vi "pop.vi"(0 "Buffer":string) -> (1 "New Buffer":string, 2 "Value":u8)   [LabVIEW 2022 SP3]
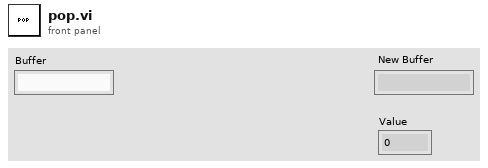
[diagram p1: front panel]
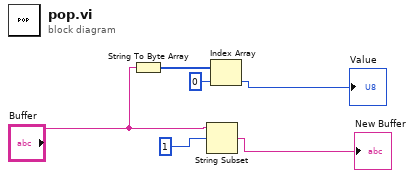
[diagram p0: block diagram]
diagram:
  n1 = String To Byte Array(string="Buffer") -> (unsigned byte array=w3:u8[])
  n2 = String Subset(string="Buffer", offset (0)=1) -> (substring=→"New Buffer":string)  [unwired: 1 in]
  n3 = Index Array(array=w3, index=0) -> (element=→"Value":u8)
